vi "Brute Force Measurment SubVI.vi"(0 "Barcodes in":string[](array[string]), 1 "Engaged Tube Ch0":refnum<vi>, 2 "Engaged Tube Ch1":refnum<vi>, 4 "BoardHandle in":T1, 5 "error in (no error)":errorcluster, 6 "Current Ch 0":refnum<vi>, 7 "Ch 0 Currents":refnum<vi>, 8 "Current Ch 1":refnum<vi>, 9 "Ch 1 Currents":refnum<vi>, 10 "Channel 0 Leak":dbl, 15 "Channel 1 Leak":dbl) -> (12 "Bool Bad 1":bool[](array[boolean]), 13 "Bool Bad 2":bool[](array[boolean]), 14 "Bad Tubes":string[](array[string]), 16 "Trip?":bool, 18 "BoardHandle out":T1, 19 "error out":errorcluster)   [LabVIEW 2020]
uses:
  <instrlib>/CAEN PSM/CAEN PSM.lvlib
panel:
  in  "User":string
  # "INPUT"
  # "OUTPUT"
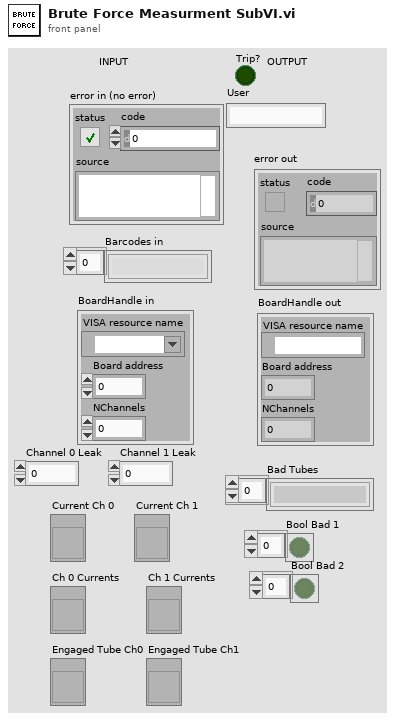
[diagram p1: front panel]
types:
  T1 = cluster{"VISA resource name":refnum<visa-resource-name>, "Board address":u8, "NChannels":u8}
  T2 = typedef "CAEN PSM.lvlib/BoardHandle.ctl" = cluster{"VISA resource name":refnum<visa-resource-name>, "Board address":i8, "NChannels":u8}
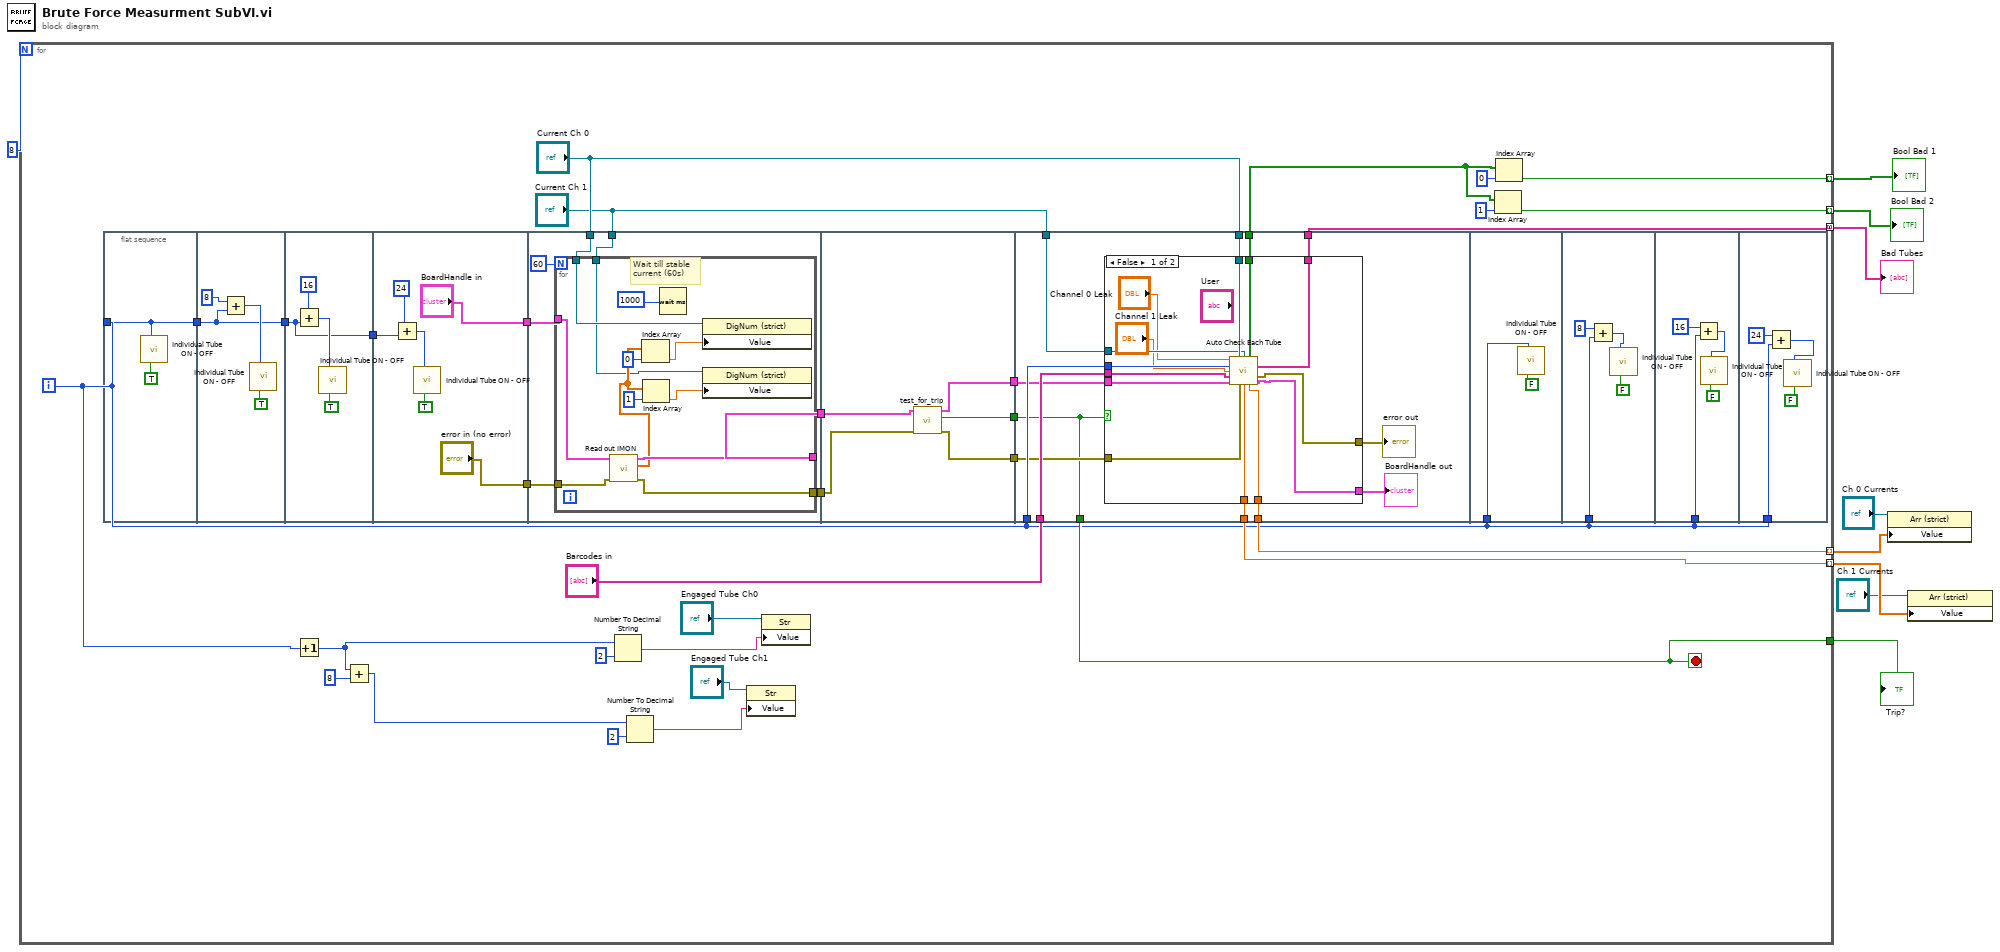
[diagram p0: block diagram]
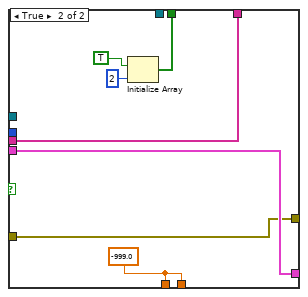
[diagram p2: hidden frame]
diagram:
  n1 = for {
    N: 8 -> [_]
    tunnel: [w38] -> w8 mode=concatenating
    tunnel: [w34] -> w7 mode=indexing
    tunnel: [w33] -> w6 mode=indexing
    tunnel: [w32] -> w4 mode=indexing
    tunnel: [w31] -> w3 mode=indexing
    tunnel: [w27] -> w1
    i -> [w11]
    stop <- w27 stop-if-true
    n2 = flat-sequence {
      tunnel: w11 -> [w42]
      tunnel: [w42] -> w41
      tunnel: w41 -> [w45]
      tunnel: [w45] -> w40
      tunnel: w40 -> [w49]
      tunnel: [w49] -> w39
      tunnel: w39 -> [w55]
      tunnel: ["BoardHandle in"] -> w25
      tunnel: ["error in (no error)"] -> w23
      tunnel: [w62] -> w26
      tunnel: w25 -> [w64]
      tunnel: [w61] -> w24
      tunnel: w23 -> [w63]
      tunnel: "Current Ch 0" -> [w60]
      tunnel: "Current Ch 1" -> [w59]
      tunnel: [w81] -> w30
      tunnel: [w80] -> w29
      tunnel: [w79] -> w28
      tunnel: w26 -> [w78]
      tunnel: w24 -> [w77]
      tunnel: w11 -> [w90]
      tunnel: [w94] -> w38
      tunnel: [w89] -> w35
      tunnel: "Barcodes in" -> [w91]
      tunnel: [w88] -> w31
      tunnel: [w87] -> w32
      tunnel: w30 -> [w86]
      tunnel: w29 -> [w85]
      tunnel: w28 -> [w84]
      tunnel: [w84] -> w27
      tunnel: "Current Ch 0" -> [w83]
      tunnel: "Current Ch 1" -> [w82]
      tunnel: w11 -> [w117]
      tunnel: w11 -> [w120]
      tunnel: w11 -> [w124]
      tunnel: w11 -> [w128]
      frame #0 {
        n3 = call "Individual Tube ON - OFF.vi"("Single Tube ON/OFF"=TRUE, "Tube #"=w42) -> ()  [unwired: 10 in]
      }
      frame #1 {
        n4 = Add(x=8, y=w45) -> (x+y=w47:i32)
        n5 = call "Individual Tube ON - OFF.vi"("Single Tube ON/OFF"=TRUE, "Tube #"=w47) -> ()  [unwired: 10 in]
      }
      frame #2 {
        n6 = Add(x=16, y=w49) -> (x+y=w51:i32)
        n7 = call "Individual Tube ON - OFF.vi"("Single Tube ON/OFF"=TRUE, "Tube #"=w51) -> ()  [unwired: 10 in]
      }
      frame #3 {
        n8 = Add(x=24, y=w55) -> (x+y=w57:i32)
        n9 = call "Individual Tube ON - OFF.vi"("Single Tube ON/OFF"=TRUE, "Tube #"=w57) -> ()  [unwired: 10 in]
      }
      frame #4 {
        n10 = for {
          N: 60 -> [_]
          tunnel: w64 -> [w76]
          tunnel: w63 -> [w75]
          tunnel: [w74] -> w62
          tunnel: [w73] -> w61
          tunnel: w60 -> [w67]
          tunnel: w59 -> [w66]
          # "Wait till stable\ncurrent (60s)"
          n11 = call <instrlib>:"Read out IMON.vi"("error in (no error)"=w75, "BoardHandle"=w76) -> ("error out"=w73:errorcluster, "IMon values (uA)"=w68:dbl[], "BoardHandle out"=w74:T2)  [unwired: 6 in, 1 out]
          n12 = Index Array(array=w68, index=0) -> (element=w72:dbl)
          n13 = Index Array(array=w68, index=1) -> (element=w71:dbl)
          n14 = Wait (ms)(milliseconds to wait=u32 1000) -> ()  [unwired: 1 out]
          n15 = property class="DigNum (strict)"(reference=w67, "Value"=w72) -> ()  [unwired: 1 in, 2 out]
          n16 = property class="DigNum (strict)"(reference=w66, "Value"=w71) -> ()  [unwired: 1 in, 2 out]
        }
      }
      frame #5 {
        n17 = call "test_for_trip.vi"("error in (no error)"=w77, "BoardHandle in"=w78) -> ("error out"=w80:errorcluster, "Trip?"=w79:bool, "BoardHandle out 3"=w81:T1)  [unwired: 7 in]
      }
      frame #6 {
        n18 = case shown="False" w84 {
          tunnel: [w108 w109] -> w94
          tunnel: [w107 w113] -> w93
          tunnel: [w106 w114] -> w92
          tunnel: w91 -> [w105 w109]
          tunnel: w90 -> [w104 _]
          tunnel: [w103 w110] -> w89
          tunnel: [w102 w115] -> w88
          tunnel: [w101 w115] -> w87
          tunnel: w86 -> [w100 w114]
          tunnel: w85 -> [w99 w113]
          tunnel: w83 -> [w98 _]
          tunnel: w82 -> [w97 _]
          frame False {
            n19 = call "Auto Check Each Tube.vi"("Ch 0 Leak"="Channel 0 Leak", "Cur Ch 0"=w98, "Cur Ch 1"=w97, "Tube #"=w104, "Ch 1 Leak"="Channel 1 Leak", "Barcodes in"=w105, "BoardHandle in"=w100, "error in (no error)"=w99) -> ("Bool Bad Tubes"=w103:bool[], "Bad Tubes"=w108:string[], "error out"=w107:errorcluster, "Channel 1 current"=w102:dbl, "Channel 0 current"=w101:dbl, "BoardHandle out"=w106:T1)  [unwired: 2 in]
          }
          frame True {
            w115 = -999.0 ("Channel 1 current")
            n20 = Initialize Array(TRUE, 2 ("dimension size")) -> (w110:bool[])
          }
        }
        "error out" <- w93
        "BoardHandle out" <- w92
      }
      frame #7 {
        n21 = call "Individual Tube ON - OFF.vi"("Single Tube ON/OFF"=FALSE, "Tube #"=w117) -> ()  [unwired: 10 in]
      }
      frame #8 {
        n22 = Add(x=8, y=w120) -> (x+y=w121:i32)
        n23 = call "Individual Tube ON - OFF.vi"("Single Tube ON/OFF"=FALSE, "Tube #"=w121) -> ()  [unwired: 10 in]
      }
      frame #9 {
        n24 = Add(x=16, y=w124) -> (x+y=w125:i32)
        n25 = call "Individual Tube ON - OFF.vi"("Single Tube ON/OFF"=FALSE, "Tube #"=w125) -> ()  [unwired: 10 in]
      }
      frame #10 {
        n26 = Add(x=24, y=w128) -> (x+y=w129:i32)
        n27 = call "Individual Tube ON - OFF.vi"("Single Tube ON/OFF"=FALSE, "Tube #"=w129) -> ()  [unwired: 10 in]
      }
    }
    n28 = Increment(x=w11) -> (x+1=w10:i32)
    n29 = Add(x=w10, y=8) -> (x+y=w15:i32)
    n30 = Number To Decimal String(number=w10, width (-)=i16 2) -> (decimal integer string=w13:string)
    n31 = Number To Decimal String(number=w15, width (-)=i16 2) -> (decimal integer string=w14:string)
    n32 = property on="Property Node" class="Str"(reference="Engaged Tube Ch1", "Value"=w14) -> ()  [unwired: 1 in, 2 out]
    n33 = property on="Property Node" class="Str"(reference="Engaged Tube Ch0", "Value"=w13) -> ()  [unwired: 1 in, 2 out]
    n34 = Index Array(array=w35, index=1) -> (element=w33:bool)
    n35 = Index Array(array=w35, index=0) -> (element=w34:bool)
  }
  "Bad Tubes" <- w8
  "Bool Bad 1" <- w7
  "Bool Bad 2" <- w6
  "Trip?" <- w1
  n36 = property class="Arr (strict)"(reference="Ch 0 Currents", "Value"=w4) -> ()  [unwired: 1 in, 2 out]
  n37 = property class="Arr (strict)"(reference="Ch 1 Currents", "Value"=w3) -> ()  [unwired: 1 in, 2 out]
